vi "PJM decoder.vi"(8 "error in (no error)":errorcluster, 11 "Bit stream in":u8[](array[numeric])) -> (0 "error out":errorcluster, 3 "output array":u8[](array[numeric]))   [LabVIEW 2019]
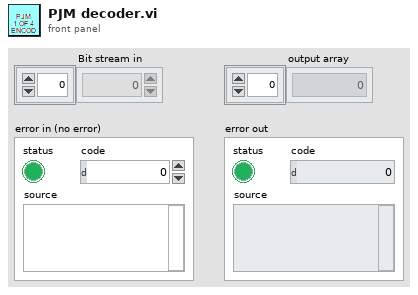
[diagram p1: front panel]
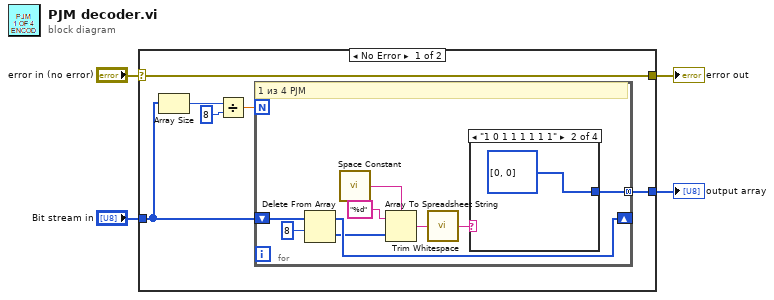
[diagram p0: block diagram]
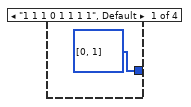
[diagram p2: hidden frame]
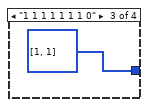
[diagram p3: hidden frame]
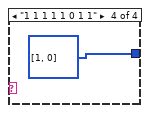
[diagram p4: hidden frame]
diagram:
  n1 = case shown="No Error" "error in (no error)" {
    selector: "error in (no error)" -> [w10 w24]
    tunnel: "Bit stream in" -> [w6 _]
    tunnel: [w10 w24] -> w2
    tunnel: [w5 _] -> w1
    frame No Error {
      n2 = Array Size(array=w6) -> (size(s)=w9:i32)
      n3 = Divide(x=w9, y=8) -> (x/y=w7:dbl)
      n4 = for {
        N: w7 -> [_]
        shift-right: [w18] -> _
        shift-left: w6 -> [w19]
        tunnel: [w11] -> w5 mode=concatenating
        # "1 из 4 PJM"
        n5 = Delete From Array(array=w19, length=8) -> (deleted portion=w16:u8[], array with subset deleted=w18:u8[])  [unwired: 1 in]
        n6 = call <vilib>:"Space Constant.vi"() -> ("String"=w12:string)
        n7 = Array To Spreadsheet String(delimiter (Tab)=w12, array=w16, 3:"%d" ("format string")) -> (spreadsheet string=w14:string)
        n8 = call <vilib>:"Trim Whitespace.vi"("string"=w14) -> ("trimmed string"=w13:string)  [unwired: 1 in]
        n9 = case shown="\"1 0 1 1 1 1 1 1\"" w13 {
          tunnel: [u8[] [0, 1] ("output array") u8[] [0, 0] ("output array") u8[] [1, 1] ("output array") u8[] [1, 0] ("output array")] -> w11
          frame "1 1 1 0 1 1 1 1", Default {
          }
          frame "1 0 1 1 1 1 1 1" {
          }
          frame "1 1 1 1 1 1 1 0" {
          }
          frame "1 1 1 1 1 0 1 1" {
          }
        }
      }
    }
    frame Error {
    }
  }
  "error out" <- w2
  "output array" <- w1
